vi "Interrupcion.vi"() -> ()   [LabVIEW 2016]
panel:
  out "Numeric Control 2":i32
  out "Numeric Control":i32
  in  "Down Button":bool
  in  "Up Button":bool
  in  "Stop Button":bool
  out "Boolean 2":bool
  in  "Boolean":bool
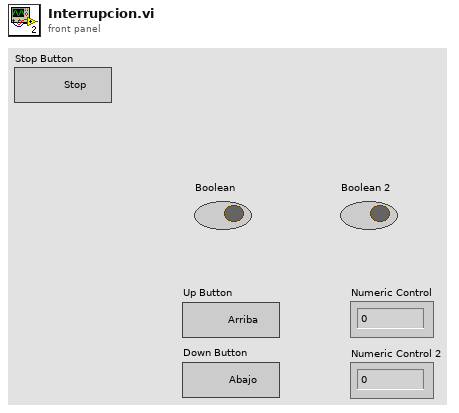
[diagram p1: front panel]
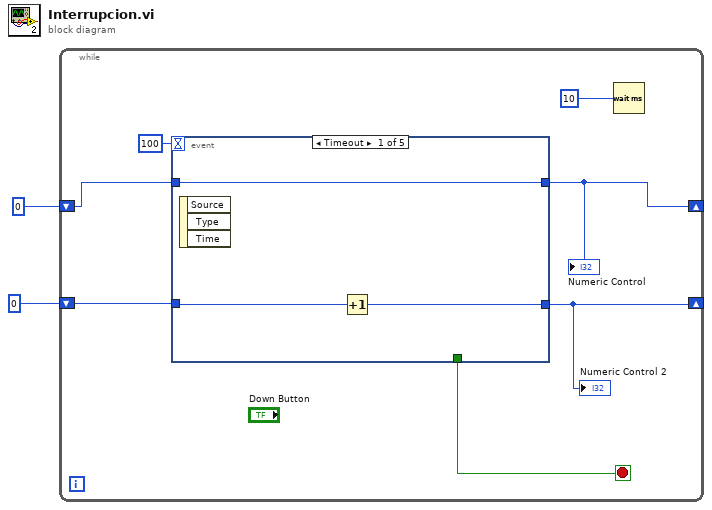
[diagram p0: block diagram]
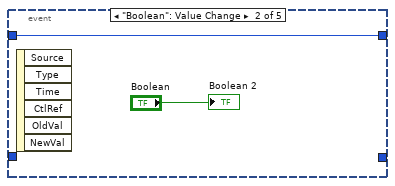
[diagram p2: hidden frame]
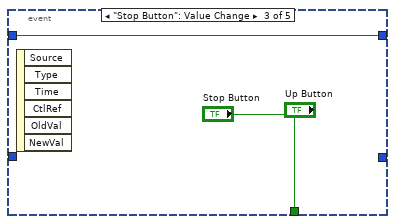
[diagram p3: hidden frame]
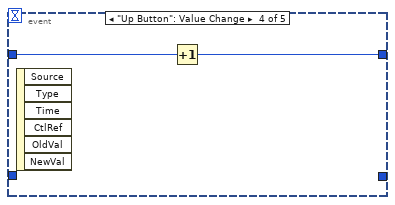
[diagram p4: hidden frame]
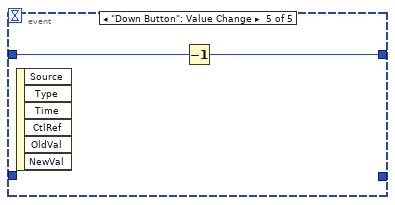
[diagram p5: hidden frame]
diagram:
  n1 = while {
    shift-right: [w6] -> _
    shift-left: 0 -> [w7]
    shift-right: [w3] -> _
    shift-left: 0 -> [w4]
    stop <- w8 stop-if-true
    n2 = event shown="[0] Timeout" {
      selector: _ -> [_ _ _ _ _]
      dyn-events: _ -> [_ _ _ _ _]
      timeout: 100 -> [_ _ _ _ _]
      tunnel: [_ _ "Stop Button" _ _] -> w8
      tunnel: w7 -> [w12 w13 w15 w18 w20]
      tunnel: [w12 w13 w15 w17 w19] -> w6
      tunnel: w4 -> [w11 _ _ _ _]
      tunnel: [w10 _ _ _ _] -> w3
      event Timeout {
        n3 = event-data() -> ()  [unwired: 1 in, 3 out]
        n4 = Increment(x=w11) -> (x+1=w10:i32)
      }
      event "Boolean": Value Change {
        n5 = event-data() -> ()  [unwired: 1 in, 6 out]
        "Boolean 2" <- "Boolean"
      }
      event "Stop Button": Value Change {
        n6 = event-data() -> ()  [unwired: 1 in, 6 out]
      }
      event "Up Button": Value Change {
        n7 = event-data() -> ()  [unwired: 1 in, 6 out]
        n8 = Increment(x=w18) -> (x+1=w17:i32)
      }
      event "Down Button": Value Change {
        n9 = event-data() -> ()  [unwired: 1 in, 6 out]
        n10 = Decrement(x=w20) -> (x-1=w19:i32)
      }
    }
    "Numeric Control" <- w6
    "Numeric Control 2" <- w3
    n11 = Wait (ms)(milliseconds to wait=u32 10) -> ()  [unwired: 1 out]
  }
